vi "MB ICPCON Registers Read WR.vi"(7 "Data Reference":T1, 8 "error in (no error)":errorcluster, 11 "N":i32) -> (0 "error out":errorcluster, 1 "Words out":u16[](array[numeric]))   [LabVIEW 2021, in "ICPCON Registers.lvlib"]
uses:
  ICPCON Registers.lvlib
  Ctl/ICPCON Data.ctl
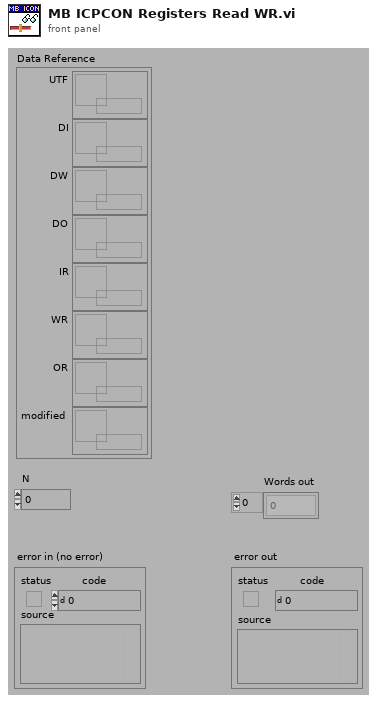
[diagram p1: front panel]
types:
  T1 = typedef "ICPCON Registers.lvlib/ICPCON Data.ctl" = cluster{"UTF":refnum<data-value>, "DI":refnum<data-value>, "DW":refnum<data-value>, "DO":refnum<data-value>, "IR":refnum<data-value>, "WR":refnum<data-value>, "OR":refnum<data-value>, "modified":refnum<data-value>}
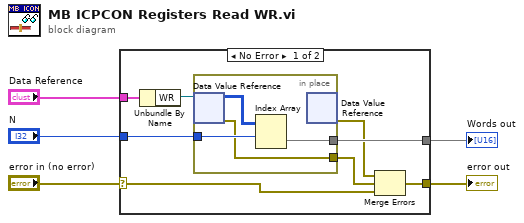
[diagram p0: block diagram]
diagram:
  n1 = case shown="No Error" "error in (no error)" {
    selector: "error in (no error)" -> [w6 w18]
    tunnel: [w10 w18] -> w5
    tunnel: [w13 _] -> w4
    tunnel: "N" -> [w12 _]
    tunnel: "Data Reference" -> [w11 _]
    frame No Error {
      n2 = Unbundle By Name(w11) -> ("WR"=w7:refnum<data-value>)
      n3 = in-place {
        in-place-border: w12 -> [w17]
        in-place-border: [w15] -> w13
        in-place-border: [w14] -> w8
        n4 = in-place-dvr #1(w7) -> (w16:u16[][], w14:errorcluster)
        n5 = Index Array(array=w16, index (row)=w17) -> (element=w15:u16[])  [unwired: 1 in]
        n6 = in-place-dvr #1() -> (w9:errorcluster)  [unwired: 1 in, 1 out]
      }
      n7 = Merge Errors(w9, w8, w6) -> (w10:errorcluster)
    }
    frame Error {
    }
  }
  "error out" <- w5
  "Words out" <- w4
